vi "50 NMEA Calc Checksum (x64-2018).vi"(0 "GPS String":string="PASHR,POS,0,07,212227.20,3018.85766,N,09747.91007,W,+00218.00,,154.51,000.12,+000.08,05.0,03.1,04.0,03.7,GM00*2B") -> (1 "Checksum Calculated":u8 format="%x", 2 "hex integer string":string)   [LabVIEW 2017]
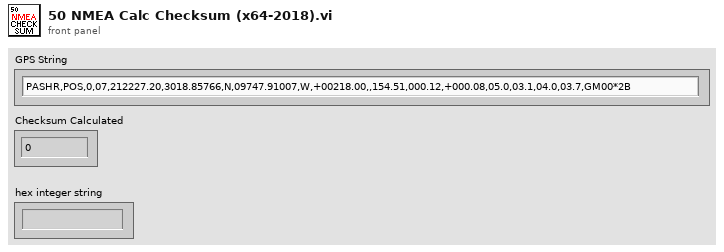
[diagram p1: front panel]
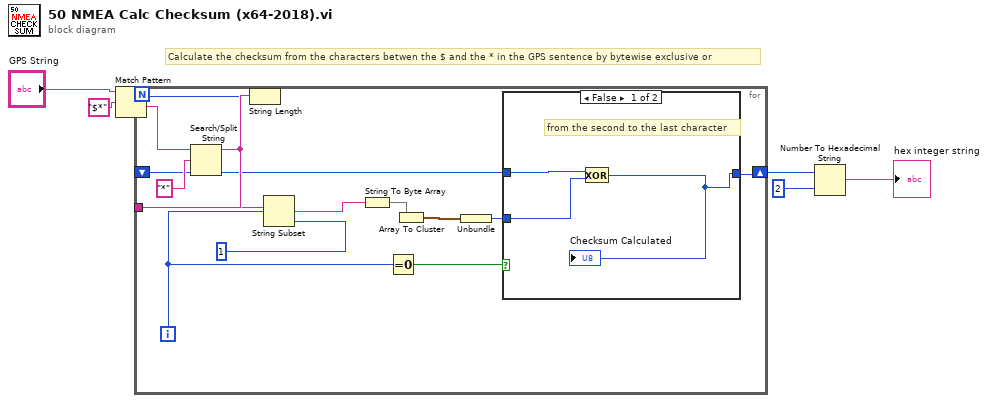
[diagram p0: block diagram]
diagram:
  # "Calculate the checksum from the characters betwen the $ and the * in the GPS sentence by bytewise exclusive or"
  n1 = Match Pattern(string="GPS String", regular expression="$*") -> (after substring=w5:string)  [unwired: 1 in, 3 out]
  n2 = Search/Split String(string=w5, search string/char (-)="*") -> (substring before match=w8:string)  [unwired: 1 in, 2 out]
  n3 = String Length(string=w8) -> (length=w7:i32)
  n4 = for {
    N: w7 -> [_]
    tunnel: w8 -> [w19]
    shift-right: [w12] -> w4
    shift-left: _ -> [w10]
    i -> [w17]
    n5 = String Subset(string=w19, offset (0)=w17, length (rest)=1) -> (substring=w14:string)
    n6 = String To Byte Array(string=w14) -> (unsigned byte array=w15:u8[])
    n7 = Equal To 0?(x=w17) -> (x = 0?=w11:bool)
    n8 = Array To Cluster(array=w15) -> (cluster=w16:cluster{"unsigned byte array[0]":u8})
    n9 = Unbundle(w16) -> ("unsigned byte array[0]"=w13:u8)
    n10 = case shown="False" w11 {
      tunnel: w13 -> [w22 w23]
      tunnel: [w20 w23] -> w12
      tunnel: w10 -> [w21 _]
      frame False {
        # "from the second to the last character"
        n11 = Exclusive Or(1:w22, 2:w21) -> (0:w20:u8)
        "Checksum Calculated" <- w20
      }
      frame True {
        # "Get the first character ready (\"P\")"
      }
    }
  }
  n12 = Number To Hexadecimal String(1:i16 2 ("width (-)"), 2:w4) -> (0:→"hex integer string":string)
